vi "Configure Spectrum Emission Mask (Reference Setup).vi"(0 "VISA resource name":refnum<visa-resource-name>, 1 "SEM Attenuator (10dB)":i32=10 min=0 max=60, 2 "SEM Attenuator Auto (1:On)":i32(ring)=1 items=["Off", "On"], 3 "SEM Couple Reference Attenuator (1:On)":i32(ring)=1 items=["Off", "On"], 5 "SEM Meas. Type (0:Integral power)":i32(ring) items=["Integral Power", "Peak Power", "Fixed"], 7 "SEM Resolution Bandwidth (3840000Hz)":dbl=3840000.0 min=1000.0 max=200000000.0, 9 "SEM Reference Power (0.00dBm)":dbl min=-200.0 max=200.0 format="%.2f", 11 "error in (no error)":errorcluster, 12 "SEM Filter Type (0:Rectangular Filter)":i32(ring) items=["Rectangular Filter", "Nyquist Filter", "Root Nyquist Filter"], 13 "SEM Ratio (0.22)":dbl=0.22 min=0.01 max=1.0 format="%.2f") -> (4 "VISA resource name out":refnum<visa-resource-name>, 15 "error out":errorcluster)   [LabVIEW 2020, in "Anritsu Signal Analyzer Series.lvlib"]
doc: "Configures the setup for reference parameter of SEM measurement settings of the spectrum analyzer."
uses:
  Anritsu Signal Analyzer Series.lvlib
panel:
  # "Hz"
  # "dBm"
  # "dB"
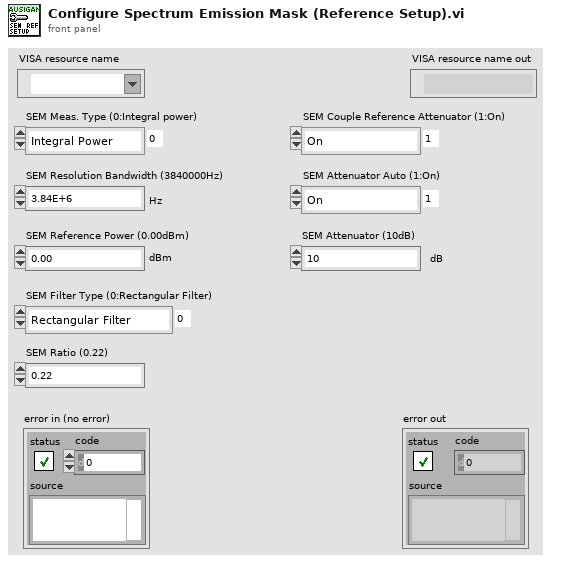
[diagram p1: front panel]
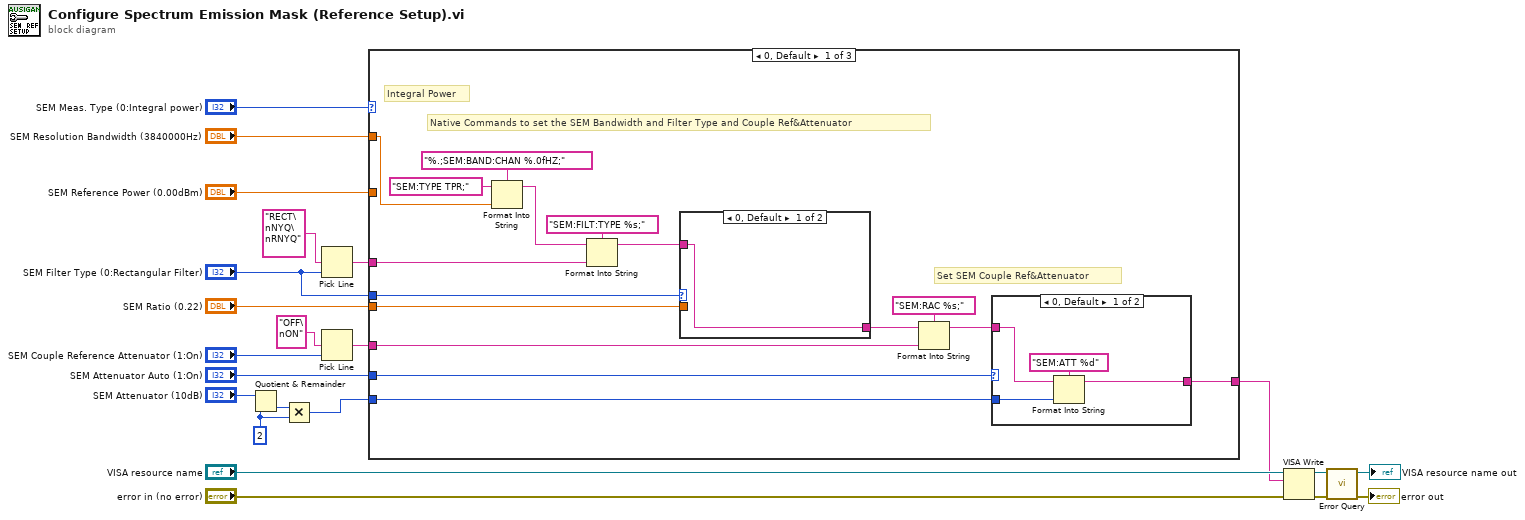
[diagram p0: block diagram]
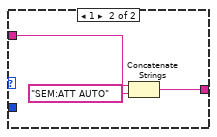
[diagram p2: hidden frame]
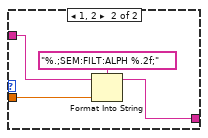
[diagram p3: hidden frame]
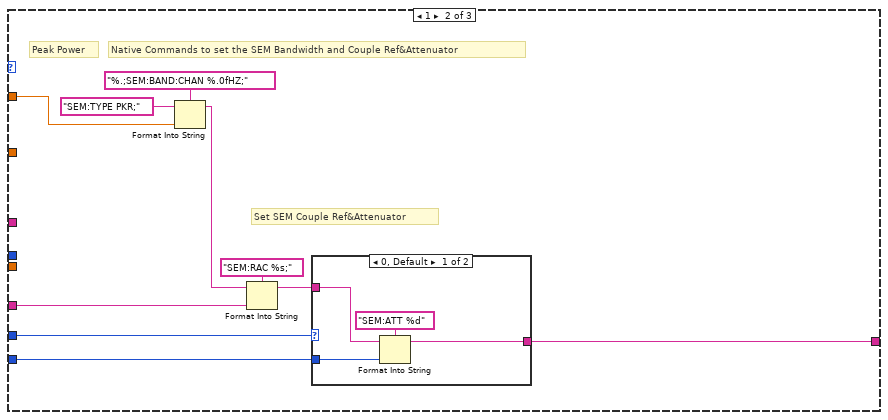
[diagram p4: hidden frame]
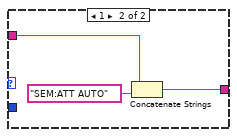
[diagram p5: hidden frame]
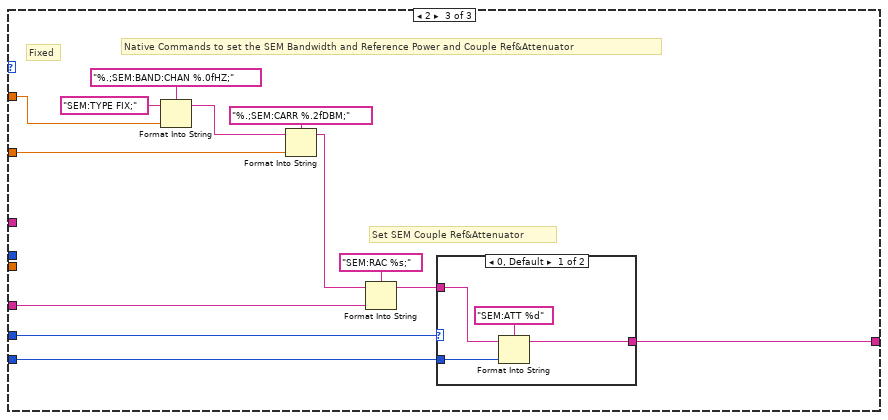
[diagram p6: hidden frame]
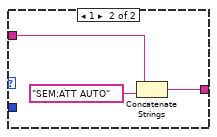
[diagram p7: hidden frame]
diagram:
  w8 = 2
  n1 = Quotient & Remainder(x="SEM Attenuator (10dB)", y=w8) -> (floor(x/y)=w7:i32)  [unwired: 1 out]
  n2 = Multiply(x=w7, y=w8) -> (x*y=w5:i32)
  n3 = Pick Line(multi-line string="RECT\nNYQ\nRNYQ" ("複数行文字列"), line index="SEM Filter Type (0:Rectangular Filter)") -> (output string=w1:string)  [unwired: 1 in]
  n4 = Pick Line(multi-line string="OFF\nON" ("複数行文字列"), line index="SEM Couple Reference Attenuator (1:On)") -> (output string=w3:string)  [unwired: 1 in]
  n5 = case shown="0, Default" "SEM Meas. Type (0:Integral power)" {
    tunnel: [w38 w51 w68] -> w6
    tunnel: "SEM Reference Power (0.00dBm)" -> [_ _ w79]
    tunnel: w1 -> [w37 _ _]
    tunnel: w3 -> [w34 w60 w78]
    tunnel: w5 -> [w30 w52 w69]
    tunnel: "SEM Ratio (0.22)" -> [w29 _ _]
    tunnel: "SEM Filter Type (0:Rectangular Filter)" -> [w28 _ _]
    tunnel: "SEM Attenuator Auto (1:On)" -> [w27 w53 w70]
    tunnel: "SEM Resolution Bandwidth (3840000Hz)" -> [w23 w57 w74]
    frame 0, Default {
      # "Native Commands to set the SEM Bandwidth and Filter Type and Couple Ref&Attenuator"
      # "Set SEM Couple Ref&Attenuator"
      # "Integral Power"
      n6 = Format Into String(format string="%.;SEM:BAND:CHAN %.0fHZ;" ("Format String"), initial string="SEM:TYPE TPR;" ("_CommandSet"), w23) -> (resulting string=w24:string)  [unwired: 1 in, 1 out]
      n7 = Format Into String(format string="SEM:FILT:TYPE %s;" ("_CommandSet"), initial string=w24, w37) -> (resulting string=w35:string)  [unwired: 1 in, 1 out]
      n8 = case shown="0, Default" w28 {
        tunnel: w35 -> [w46 w49]
        tunnel: [w46 w48] -> w33
        tunnel: w29 -> [_ w47]
        frame 0, Default {
        }
        frame 1, 2 {
          n9 = Format Into String(format string="%.;SEM:FILT:ALPH %.2f;" ("Format String"), initial string=w49, w47) -> (resulting string=w48:string)  [unwired: 1 in, 1 out]
        }
      }
      n10 = Format Into String(format string="SEM:RAC %s;" ("_CommandSet"), initial string=w33, w34) -> (resulting string=w31:string)  [unwired: 1 in, 1 out]
      n11 = case shown="0, Default" w27 {
        tunnel: [w42 w44] -> w38
        tunnel: w31 -> [w41 w45]
        tunnel: w30 -> [w39 _]
        frame 0, Default {
          n12 = Format Into String(format string="SEM:ATT %d" ("Format String"), initial string=w41, w39) -> (resulting string=w42:string)  [unwired: 1 in, 1 out]
        }
        frame 1 {
          n13 = Concatenate Strings(w45, "SEM:ATT AUTO" ("Format String")) -> (w44:string)
        }
      }
    }
    frame 1 {
      # "Native Commands to set the SEM Bandwidth and Couple Ref&Attenuator"
      # "Set SEM Couple Ref&Attenuator"
      # "Peak Power"
      n14 = Format Into String(format string="%.;SEM:BAND:CHAN %.0fHZ;" ("Format String"), initial string="SEM:TYPE PKR;" ("_CommandSet"), w57) -> (resulting string=w55:string)  [unwired: 1 in, 1 out]
      n15 = Format Into String(format string="SEM:RAC %s;" ("_CommandSet"), initial string=w55, w60) -> (resulting string=w54:string)  [unwired: 1 in, 1 out]
      n16 = case shown="0, Default" w53 {
        tunnel: [w64 w66] -> w51
        tunnel: w54 -> [w63 w67]
        tunnel: w52 -> [w61 _]
        frame 0, Default {
          n17 = Format Into String(format string="SEM:ATT %d" ("Format String"), initial string=w63, w61) -> (resulting string=w64:string)  [unwired: 1 in, 1 out]
        }
        frame 1 {
          n18 = Concatenate Strings(w67, "SEM:ATT AUTO" ("Format String")) -> (w66:string)
        }
      }
    }
    frame 2 {
      # "Native Commands to set the SEM Bandwidth and Reference Power and Couple Ref&Attenuator"
      # "Set SEM Couple Ref&Attenuator"
      # "Fixed"
      n19 = Format Into String(format string="%.;SEM:BAND:CHAN %.0fHZ;" ("Format String"), initial string="SEM:TYPE FIX;" ("_CommandSet"), w74) -> (resulting string=w73:string)  [unwired: 1 in, 1 out]
      n20 = Format Into String(format string="%.;SEM:CARR %.2fDBM;" ("Format String"), initial string=w73, w79) -> (resulting string=w76:string)  [unwired: 1 in, 1 out]
      n21 = Format Into String(format string="SEM:RAC %s;" ("_CommandSet"), initial string=w76, w78) -> (resulting string=w71:string)  [unwired: 1 in, 1 out]
      n22 = case shown="0, Default" w70 {
        tunnel: [w84 w86] -> w68
        tunnel: w71 -> [w83 w87]
        tunnel: w69 -> [w81 _]
        frame 0, Default {
          n23 = Format Into String(format string="SEM:ATT %d" ("Format String"), initial string=w83, w81) -> (resulting string=w84:string)  [unwired: 1 in, 1 out]
        }
        frame 1 {
          n24 = Concatenate Strings(w87, "SEM:ATT AUTO" ("Format String")) -> (w86:string)
        }
      }
    }
  }
  n25 = VISA Write(VISA resource name="VISA resource name", write buffer=w6, error in (no error)="error in (no error)") -> (VISA resource name out=w9:refnum<visa-resource-name>, error out=w10:errorcluster)  [unwired: 1 out]
  n26 = call "Error Query.vi"("error in (no error)"=w10, "VISA resource name"=w9) -> ("error out"=→"error out":errorcluster, "VISA resource name out"=→"VISA resource name out":refnum<visa-resource-name>)  [unwired: 6 in, 2 out]
